vi "MiPS_safe_mode.vi"(4 "handle_shim_relay_in":u64, 5 "ref_big_msg":refnum<vi>, 6 "ref_relay_msg":refnum<vi>, 7 "ISOBUS address":T4, 8 "error in":errorcluster, 9 "ref_relay_status":refnum<vi>, 10 "ref_timeout_slider":refnum<vi>, 11 "ref_in":T1) -> (0 "error out":errorcluster, 1 "handle_shim_relay_out":u64, 3 "ref_out":T1)   [LabVIEW 2019]
uses:
  Mercury iXX Modules/Public/Controls/ISOBus Address.ctl
  Mercury iXX Modules/Public/Controls/Mercury Reference.ctl
  Mercury iXX Modules/Public/Controls/Comms Transport Layer.ctl
  Mercury iXX Modules/Private/Controls/Query Dynamic Reference.ctl
  Mercury iXX Modules/Public/Libraries/Magnet/Controls/Switch Heater.ctl
  Mercury iXX Modules/Public/Libraries/Magnet/Signals/Set/Switch Heater No Check (Set).vi
  Mercury iXX Modules/Public/Libraries/Magnet.lvlib
  Mercury iXX Modules/Mercury iXX.lvlib
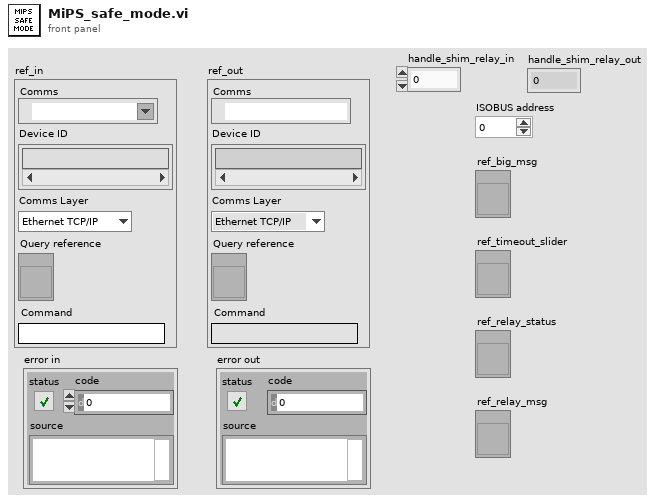
[diagram p1: front panel]
types:
  T1 = typedef "Mercury iXX.lvlib/Mercury Reference.ctl" = cluster{"Comms":refnum<visa-resource-name>, "Device ID":string[], "Comms Layer":T2, "Command":string, "Query reference":T3}
  T2 = typedef "Mercury iXX.lvlib/Comms Transport Layer.ctl" = enum16{"Ethernet TCP/IP", "USB", "ISOBus - RS-232", "GPIB"}
  T3 = typedef "Mercury iXX.lvlib/Query Dynamic Reference.ctl" = refnum<vi>
  T4 = typedef "Mercury iXX.lvlib/ISOBus Address.ctl" = i32
  T5 = typedef "Mercury iXX.lvlib/Magnet.lvlib/Switch Heater.ctl" = string
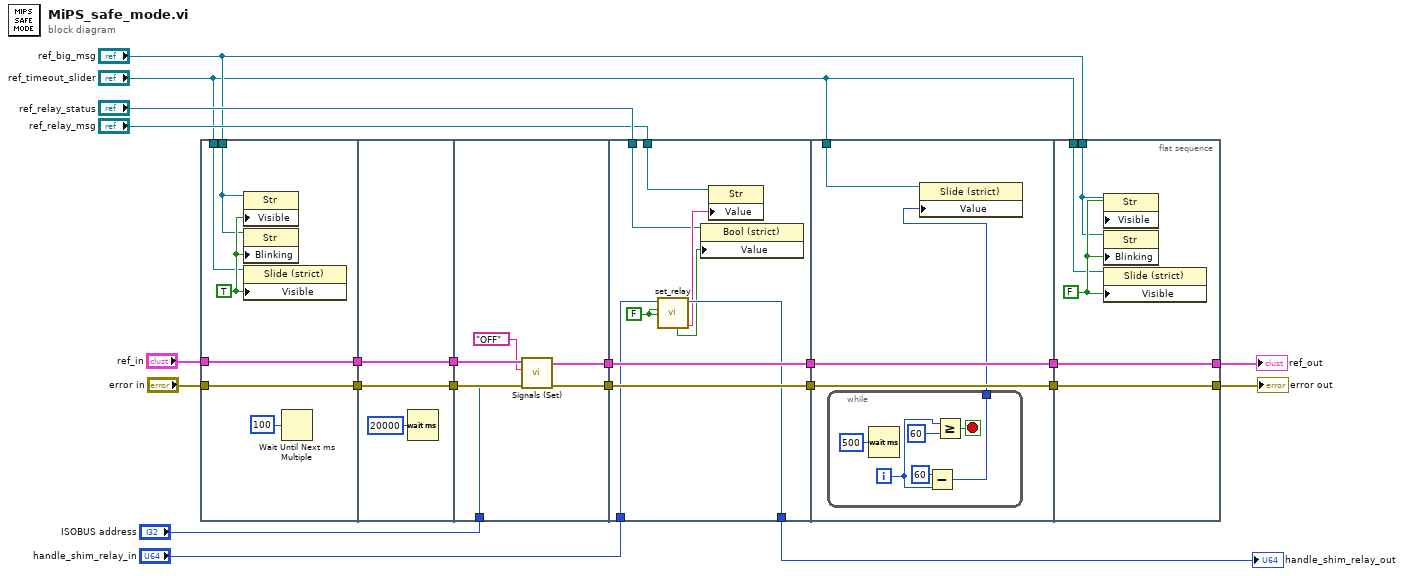
[diagram p0: block diagram]
diagram:
  n1 = flat-sequence {
    tunnel: [w27] -> w21
    tunnel: "ref_in" -> [w27]
    tunnel: [w25] -> w20
    tunnel: "error in" -> [w25]
    tunnel: "ref_big_msg" -> [w23]
    tunnel: "ref_timeout_slider" -> [w22]
    tunnel: w21 -> [w30]
    tunnel: [w30] -> w19
    tunnel: w20 -> [w29]
    tunnel: [w29] -> w18
    tunnel: w19 -> [w36]
    tunnel: w18 -> [w34]
    tunnel: [w35] -> w17
    tunnel: [w33] -> w16
    tunnel: "ISOBUS address" -> [w32]
    tunnel: w17 -> [w45]
    tunnel: [w45] -> w15
    tunnel: w16 -> [w44]
    tunnel: [w44] -> w14
    tunnel: "handle_shim_relay_in" -> [w43]
    tunnel: [w41] -> w11
    tunnel: "ref_relay_status" -> [w38]
    tunnel: "ref_relay_msg" -> [w37]
    tunnel: w15 -> [w49]
    tunnel: w14 -> [w48]
    tunnel: [w49] -> w13
    tunnel: [w48] -> w12
    tunnel: "ref_timeout_slider" -> [w47]
    tunnel: [w59] -> w7
    tunnel: [w60] -> w5
    tunnel: w13 -> [w60]
    tunnel: w12 -> [w59]
    tunnel: "ref_timeout_slider" -> [w57]
    tunnel: "ref_big_msg" -> [w56]
    frame #0 {
      w24 = TRUE ("Visible")
      n2 = property on="Property Node" class="Str"(reference=w23, "Visible"=w24) -> ()  [unwired: 1 in, 2 out]
      n3 = property on="Property Node" class="Str"(reference=w23, "Blinking"=w24) -> ()  [unwired: 1 in, 2 out]
      n4 = property on="Property Node" class="Slide (strict)"(reference=w22, "Visible"=w24) -> ()  [unwired: 1 in, 2 out]
      n5 = Wait Until Next ms Multiple(millisecond multiple=u32 100) -> ()  [unwired: 1 out]
    }
    frame #1 {
      n6 = Wait (ms)(milliseconds to wait=u32 20000) -> ()  [unwired: 1 out]
    }
    frame #2 {
      n7 = call-poly "Signals (Set).vi"("ISOBUS address"=w32, "error in"=w34, "Set Switch Heater"=T5 "OFF", "Mercury Reference In"=w36) -> ("error out"=w33:errorcluster, "Mercury Reference Out"=w35:T1)  [unwired: 4 in, 2 out]
    }
    frame #3 {
      w42 = FALSE ("ch_1")
      n8 = call "set_relay.vi"("ch_2"=w42, "ch_1"=w42, "Handle"=w43) -> ("message"=w39:string, "Handle_out"=w41:u64, "status"=w40:bool)  [unwired: 4 in, 2 out]
      n9 = property class="Bool (strict)"(reference=w38, "Value"=w40) -> ()  [unwired: 1 in, 2 out]
      n10 = property class="Str"(reference=w37, "Value"=w39) -> ()  [unwired: 1 in, 2 out]
    }
    frame #4 {
      n11 = while {
        tunnel: [w50] -> w46
        i -> [w52]
        stop <- w54 stop-if-true
        n12 = Wait (ms)(milliseconds to wait=u32 500) -> ()  [unwired: 1 out]
        n13 = Subtract(x=60, y=w52) -> (x-y=w50:i32)
        n14 = Greater Or Equal?(x=w52, y=60) -> (x >= y?=w54:bool)
      }
      n15 = property class="Slide (strict)"(reference=w47, "Value"=w46) -> ()  [unwired: 1 in, 2 out]
    }
    frame #5 {
      w58 = FALSE ("Visible")
      n16 = property on="Property Node" class="Str"(reference=w56, "Visible"=w58) -> ()  [unwired: 1 in, 2 out]
      n17 = property on="Property Node" class="Str"(reference=w56, "Blinking"=w58) -> ()  [unwired: 1 in, 2 out]
      n18 = property on="Property Node" class="Slide (strict)"(reference=w57, "Visible"=w58) -> ()  [unwired: 1 in, 2 out]
    }
  }
  "handle_shim_relay_out" <- w11
  "error out" <- w7
  "ref_out" <- w5
